vi "WPI_CameraDirect Read from Laptop.vi"(6 "Camera Settings 2":T3={"Exposure"=enum."Auto", "Exposure (%)"=50.0, "Brightness"=50, "White Balance"=enum."Auto", "Color Temp (K)"=0.0} {"Brightness" min=0 max=100}, 7 "Operation":enum16{"Read", "Reopen", "Close"}(ring), 8 "error in":errorcluster, 9 "Camera Settings":T5={"fps"=30, "compression"=30, "Image Size"=enum."320x240", "Config Shown"=FALSE}, 10 "Image":T4, 11 "address":string="10.te.am.11") -> (0 "error out":errorcluster, 2 "Image Out":T4)   [LabVIEW 2017]
doc: "This VI is intended for testing, examples, and demos. It assumes the camera is directly accssible from the computer and not the robot. It retrieves an image from either a USB or IP Axis camera.\n\nThis software is licensed. Open the labview\\readme\\WPI Robotics Library Open Source License.txt file for more information."
uses:
  <vilib>/picture/picture.llb/imagedata.ctl
  <vilib>/vision/driver/NI_Vision_Acquisition_Software.lvlib
  <vilib>/Rock Robotics/WPI/Camera/WPI_CameraDevRef.ctl
  <vilib>/Rock Robotics/WPI/Camera/WPI_CameraImageSize.ctl
  <vilib>/Rock Robotics/WPI/Camera/WPI_CameraSettings Read MJPG.ctl
  <vilib>/Rock Robotics/WPI/Camera/WPI_CameraRegistryActions.ctl
  <vilib>/Rock Robotics/WPI/Camera/WPI_CameraWhite Balance Values.ctl
  <vilib>/Rock Robotics/WPI/Camera/WPI_CameraExposure Values.ctl
  <vilib>/vision/Image Controls.llb/IMAQ Image.ctl
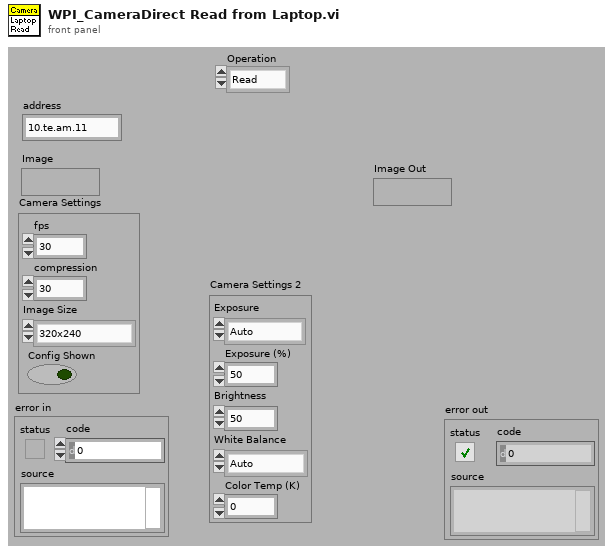
[diagram p1: front panel]
types:
  T1 = typedef "WPI_CameraExposure Values.ctl" = enum16{"Auto", "Flicker-free 50 Hz", "Flicker-free 60 Hz", "Hold current", "Custom"}
  T2 = typedef "WPI_CameraWhite Balance Values.ctl" = enum16{"Auto", "Fixed indoor", "Fixed outdoor 1", "Fixed outdoor 2", "Fixed fluorescent 1", "Fixed fluorescent 2", "Hold current", "Custom"}
  T3 = cluster{"Exposure":T1, "Exposure (%)":dbl, "Brightness":i32, "White Balance":T2, "Color Temp (K)":dbl}
  T4 = typedef "IMAQ Image.ctl" = refnum<image>
  T5 = typedef "WPI_CameraSettings Read MJPG.ctl" = cluster{"fps":i32, "compression":i32, "Image Size":T6, "Config Shown":bool}
  T6 = typedef "WPI_CameraImageSize.ctl" = enum16{"640x480", "320x240", "160x120", "Custom"}
  T7 = typedef "WPI_CameraDevRef.ctl" = cluster{"Camera Address":string, "CameraStatus":errorcluster}
  T8 = typedef "WPI_CameraRegistryActions.ctl" = enum16{"Open", "Close"}
  T9 = typedef "IMAQdx.ctl" = refnum<k21>
  T10 = cluster{"fps":bool, "compression":bool, "Image Size":bool, "Config Shown":bool}
  T11 = cluster{"Exposure":bool, "Exposure (%)":bool, "Brightness":bool, "White Balance":bool, "Color Temp (K)":bool}
  T12 = typedef "imagedata.ctl" = cluster{"image type":i32, "image depth":i32, "image":u8[], "mask":u8[], "colors":u32[], "Rectangle":cluster{"left":i16, "top":i16, "right":i16, "bottom":i16}}
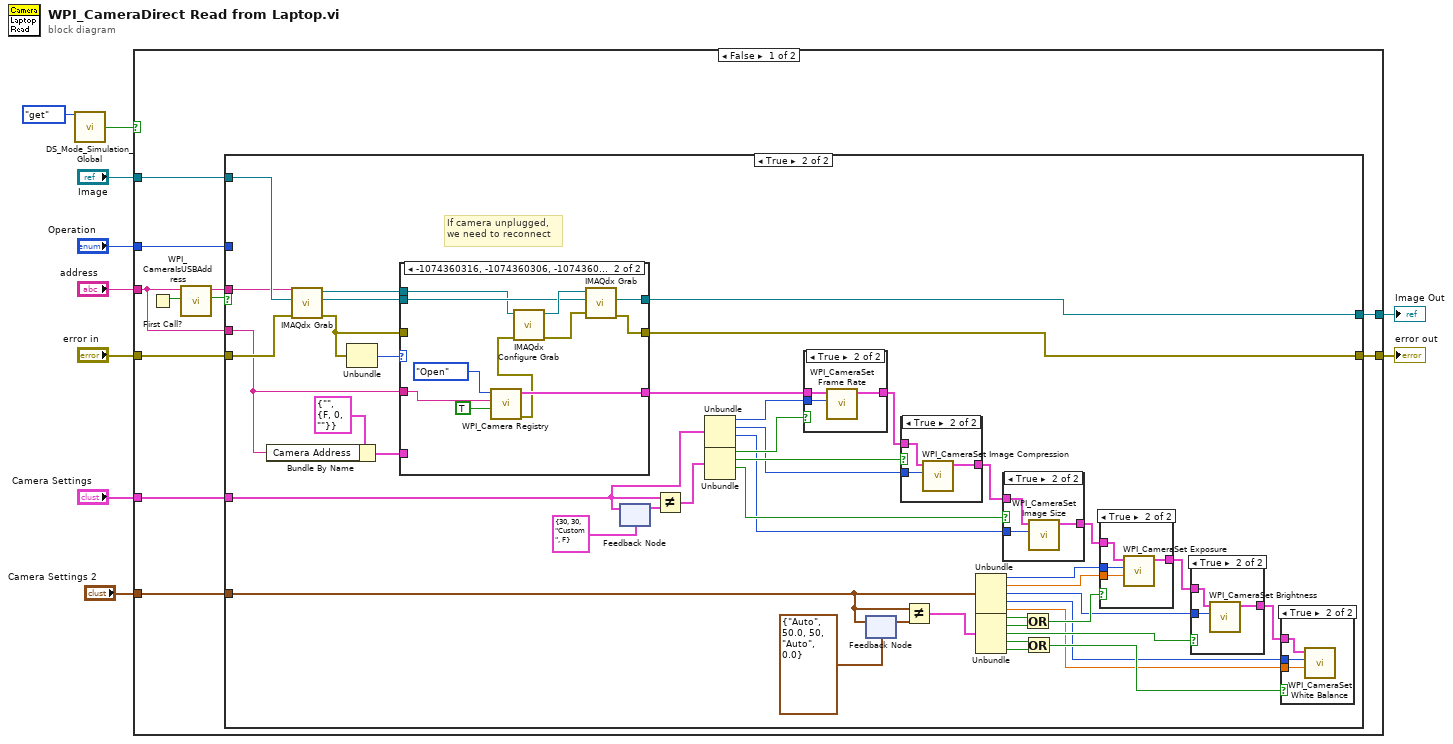
[diagram p0: block diagram]
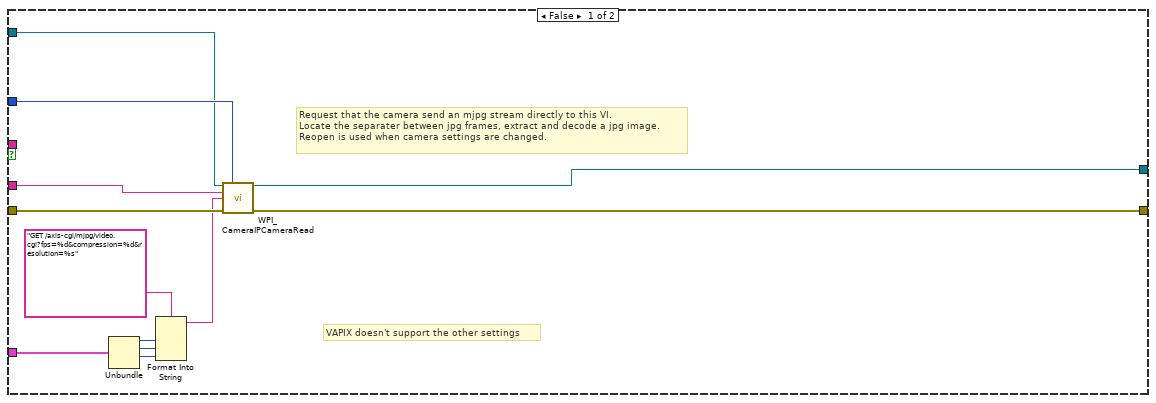
[diagram p2: hidden frame]
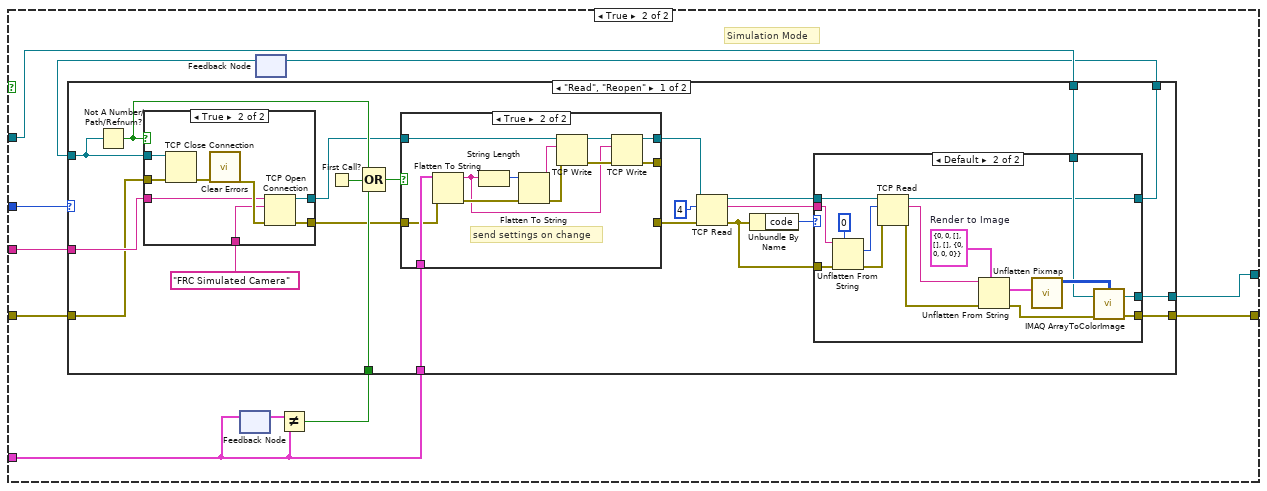
[diagram p10: hidden frame]
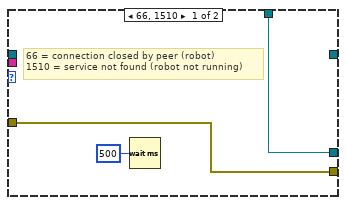
[diagram p12: hidden frame]
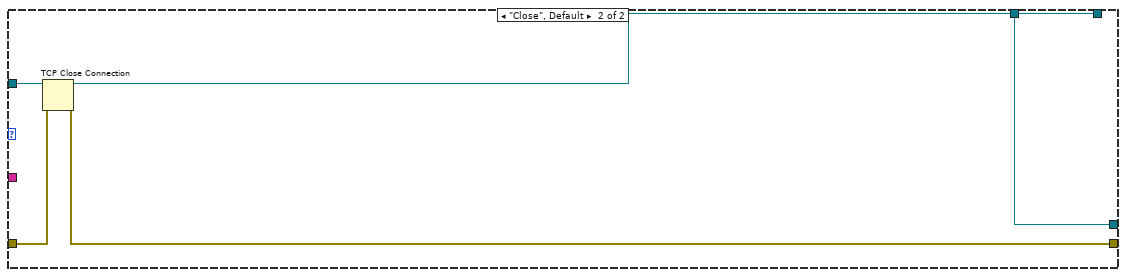
[diagram p14: hidden frame]
diagram:
  n1 = call <vilib>:"DS_Mode_Simulation_Global.vi"("menu"=enum16{"set", "get"}."get") -> ("simulated? out"=w5:bool)  [unwired: 13 in, 1 out]
  n2 = case shown="False" w5 {
    tunnel: "error in" -> [w21 w124]
    tunnel: "address" -> [w15 w125]
    tunnel: [w20 w123] -> w8
    tunnel: [w19 w122] -> w3
    tunnel: "Operation" -> [w18 w120]
    tunnel: "Image" -> [w17 w121]
    tunnel: "Camera Settings" -> [w16 w117]
    tunnel: "Camera Settings 2" -> [w11 _]
    frame False {
      n3 = First Call?() -> (First Call?: T/F=w12:bool)
      n4 = call <vilib>:"WPI_CameraIsUSBAddress.vi"("Enumerate?"=w12, "Camera Address In"=w15) -> ("USB?"=w14:bool, "Camera Address Out"=w13:string)  [unwired: 7 in, 1 out]
      n5 = case shown="True" w14 {
        tunnel: w21 -> [w31 w73]
        tunnel: w15 -> [w30 w55]
        tunnel: [w28 w70] -> w20
        tunnel: [w29 w71] -> w19
        tunnel: w18 -> [w33 _]
        tunnel: w17 -> [w32 w74]
        tunnel: w16 -> [w27 w66]
        tunnel: w13 -> [_ w58]
        tunnel: w11 -> [_ w34]
        frame False {
          # "VAPIX doesn't support the other settings"
          # "Request that the camera send an mjpg stream directly to this VI.\nLocate the separater between jpg frames, extract and decode a jpg image.\nReopen is used when camera settings are changed."
          n6 = Unbundle(w27) -> ("fps"=w24:i32, "compression"=w23:i32, "Image Size"=w22:T6)  [unwired: 1 out]
          n7 = Format Into String(format string="GET /axis-cgi/mjpg/video.cgi?fps=%d&compression=%d&resolution=%s", w24, w23, w22) -> (resulting string=w25:string)  [unwired: 2 in, 1 out]
          n8 = call <vilib>:"WPI_CameraIPCameraRead.vi"("Refnum in"=w32, "Operation"=w33, "address"=w30, "cgi string"=w25, "error in (no error)"=w31) -> ("Refnum out"=w28:T4, "error out"=w29:errorcluster)  [unwired: 6 in, 3 out]
        }
        frame True {
          # "If camera unplugged,\nwe need to reconnect"
          n9 = Bundle By Name(cluster=T7 {"Camera Address"="", "CameraStatus"={"status"=FALSE, "code"=0, "source"=""}} ("CameraDevRef"), "Camera Address"=w55) -> (w54:T7)
          n10 = call <vilib>:"IMAQdx Grab.vi"("error in"=w73, "Image In"=w74, "Session In"=w58) -> ("error out"=w72:errorcluster, "Image Out"=w75:T4, "Session Out"=w76:T9)  [unwired: 5 in, 1 out]
          n11 = Unbundle(w72) -> ("code"=w77:i32)  [unwired: 2 out]
          n12 = case shown="-1074360316, -1074360306, -1074360293" w77 {
            tunnel: [w103 w114] -> w71
            tunnel: w75 -> [w104 w111]
            tunnel: [w104 w112] -> w70
            tunnel: w76 -> [_ w106]
            tunnel: w72 -> [w103 _]
            tunnel: w55 -> [_ w108]
            tunnel: [w102 w110] -> w53
            tunnel: w54 -> [w102 _]
            frame 0, Default {
            }
            frame -1074360316, -1074360306, -1074360293 {
              n13 = call <vilib>:"WPI_Camera Registry.vi"(9:TRUE ("Disallow Simulation"), "Camera Address"=w108, "Action"=WPI_CameraRegistryActions."Open" ("Enum")) -> ("error out"=w105:errorcluster, "CameraDevRef"=w110:T7)  [unwired: 7 in]
              n14 = call <vilib>:"IMAQdx Configure Grab.vi"("error in"=w105, "Session In"=w106) -> ("error out"=w115:errorcluster, "Session Out"=w113:T9)  [unwired: 8 in]
              n15 = call <vilib>:"IMAQdx Grab.vi"("error in"=w115, "Image In"=w111, "Session In"=w113) -> ("error out"=w114:errorcluster, "Image Out"=w112:T4)  [unwired: 5 in, 2 out]
            }
          }
          n16 = feedback #1(T5 {"fps"=30, "compression"=30, "Image Size"=enum."Custom", "Config Shown"=FALSE} ("Camera Settings")) -> (w69:T5)
          n17 = feedback-in #1(w66) -> ()
          n18 = Not Equal?(x=w66, y=w69) -> (x != y?=w68:T10)
          n19 = Unbundle(w66) -> ("fps"=w61:i32, "compression"=w62:i32, "Image Size"=w63:T6)  [unwired: 1 out]
          n20 = Unbundle(w68) -> ("fps"=w67:bool, "compression"=w65:bool, "Image Size"=w64:bool)  [unwired: 1 out]
          n21 = case shown="True" w67 {
            tunnel: w61 -> [_ w101]
            tunnel: w53 -> [w98 w100]
            tunnel: [w98 w99] -> w60
            frame False {
            }
            frame True {
              n22 = call <vilib>:"WPI_CameraSet Frame Rate.vi"("Frame Rate (fps)"=w101, "CameraDevRef"=w100) -> ("CameraDevRef Out"=w99:T7)  [unwired: 8 in, 1 out]
            }
          }
          n23 = feedback #2(T3 {"Exposure"=enum."Auto", "Exposure (%)"=50.0, "Brightness"=50, "White Balance"=enum."Auto", "Color Temp (K)"=0.0} ("Camera Settings 2")) -> (w51:T3)
          n24 = feedback-in #2(w34) -> ()
          n25 = case shown="True" w65 {
            tunnel: w62 -> [_ w97]
            tunnel: w60 -> [w94 w96]
            tunnel: [w94 w95] -> w59
            frame False {
            }
            frame True {
              n26 = call <vilib>:"WPI_CameraSet Image Compression.vi"("Compression"=w97, "CameraDevRef"=w96) -> ("CameraDevRef Out"=w95:T7)  [unwired: 8 in, 1 out]
            }
          }
          n27 = Not Equal?(x=w34, y=w51) -> (x != y?=w50:T11)
          n28 = Unbundle(w34) -> ("Exposure"=w45:T1, "Exposure (%)"=w44:dbl, "Brightness"=w42:i32, "White Balance"=w36:T2, "Color Temp (K)"=w35:dbl)
          n29 = Unbundle(w50) -> ("Exposure"=w48:bool, "Exposure (%)"=w47:bool, "Brightness"=w41:bool, "White Balance"=w39:bool, "Color Temp (K)"=w38:bool)
          n30 = case shown="True" w64 {
            tunnel: w63 -> [_ w93]
            tunnel: w59 -> [w90 w92]
            tunnel: [w90 w91] -> w49
            frame False {
            }
            frame True {
              n31 = call <vilib>:"WPI_CameraSet Image Size.vi"("Image Size"=w93, "CameraDevRef"=w92) -> ("CameraDevRef Out"=w91:T7)  [unwired: 8 in, 1 out]
            }
          }
          n32 = Or(x=w48, y=w47) -> (x .or. y?=w46:bool)
          n33 = Or(x=w39, y=w38) -> (x .or. y?=w37:bool)
          n34 = case shown="True" w46 {
            tunnel: w49 -> [w85 w89]
            tunnel: [w85 w88] -> w43
            tunnel: w45 -> [_ w87]
            tunnel: w44 -> [_ w86]
            frame False {
            }
            frame True {
              n35 = call <vilib>:"WPI_CameraSet Exposure.vi"("Exposure (%)"=w86, "Exposure"=w87, "CameraDevRef"=w89) -> ("CameraDevRef Out"=w88:T7)  [unwired: 7 in, 1 out]
            }
          }
          n36 = case shown="True" w41 {
            tunnel: w43 -> [w81 w84]
            tunnel: [w81 w83] -> w40
            tunnel: w42 -> [_ w82]
            frame False {
            }
            frame True {
              n37 = call <vilib>:"WPI_CameraSet Brightness.vi"("Brightness"=w82, "CameraDevRef"=w84) -> ("CameraDevRef Out"=w83:T7)  [unwired: 8 in, 1 out]
            }
          }
          n38 = case shown="True" w37 {
            tunnel: w40 -> [_ w80]
            tunnel: w36 -> [_ w79]
            tunnel: w35 -> [_ w78]
            frame False {
            }
            frame True {
              n39 = call <vilib>:"WPI_CameraSet White Balance.vi"("Color Temp (K)"=w78, "White Balance"=w79, "CameraDevRef"=w80) -> ()  [unwired: 7 in, 2 out]
            }
          }
        }
      }
    }
    frame True {
      # "Simulation Mode"
      n40 = feedback-in #3(w117) -> ()
      n41 = feedback #3() -> (w118:T5)  [unwired: 1 in]
      n42 = feedback #4() -> (w126:refnum<k5>)  [unwired: 1 out]
      n43 = Not Equal?(x=w118, y=w117) -> (x != y?=w116:bool)
      n44 = case shown="\"Read\", \"Reopen\"" w120 {
        tunnel: w126 -> [w148 w196]
        tunnel: w125 -> [w147 _]
        tunnel: w124 -> [w146 w195]
        tunnel: [w145 w193] -> w123
        tunnel: [w138 w194] -> w122
        tunnel: w121 -> [w144 w193]
        tunnel: w117 -> [w131 _]
        tunnel: [w139 w192] -> w119
        tunnel: w116 -> [w135 _]
        frame "Read", "Reopen" {
          n45 = Not A Number/Path/Refnum?(number/path/refnum=w148) -> (NaN/Path/Refnum?=w134:bool)
          n46 = case shown="True" w134 {
            tunnel: w148 -> [w183 w191]
            tunnel: w147 -> [_ w185]
            tunnel: [w183 w188] -> w133
            tunnel: w146 -> [w182 w187]
            tunnel: [w182 w186] -> w130
            tunnel: "FRC Simulated Camera" ("service name") -> [_ w184]
            frame False {
            }
            frame True {
              n47 = TCP Close Connection(connection ID=w191, error in (no error)=w187) -> (error out=w190:errorcluster)  [unwired: 2 out]
              n48 = call <vilib>:"Clear Errors.vi"("error in (no error)"=w190) -> ("error out"=w189:errorcluster)  [unwired: 1 in, 5 out]
              n49 = TCP Open Connection(address=w185, remote port or service name=w184, error in (no error)=w189) -> (connection ID=w188:refnum<k5>, error out=w186:errorcluster)  [unwired: 2 in]
            }
          }
          n50 = First Call?() -> (First Call?: T/F=w137:bool)
          n51 = Compound Arithmetic op=OR(w134, w137, w135) -> (w136:bool)
          n52 = case shown="True" w136 {
            tunnel: w133 -> [w150 w162]
            tunnel: w131 -> [_ w160]
            tunnel: [w150 w153] -> w132
            tunnel: w130 -> [w149 w152]
            tunnel: [w149 _] -> w129
            tunnel: [_ w151] -> _
            frame False {
            }
            frame True {
              # "send settings on change"
              n53 = Flatten To String(anything=w160, error in (no error)=w152) -> (data string=w154:string, error out=w156:errorcluster)  [unwired: 2 in, 1 out]
              n54 = String Length(string=w154) -> (length=w161:i32)
              n55 = Flatten To String(anything=w161, error in (no error)=w156) -> (data string=w159:string, error out=w157:errorcluster)  [unwired: 2 in, 1 out]
              n56 = TCP Write(connection ID=w162, data in=w159, error in (no error)=w157) -> (connection ID out=w155:refnum<k5>, error out=w158:errorcluster)  [unwired: 1 in, 1 out]
              n57 = TCP Write(connection ID=w155, data in=w154, error in (no error)=w158) -> (connection ID out=w153:refnum<k5>, error out=w151:errorcluster)  [unwired: 1 in, 1 out]
            }
          }
          n58 = TCP Read(connection ID=w132, bytes to read=4, error in (no error)=w129) -> (connection ID out=w141:refnum<k5>, data out=w142:string, error out=w128:errorcluster)  [unwired: 1 in, 1 out]
          n59 = Unbundle By Name(w128) -> ("code"=w140:i32)
          n60 = case shown="Default" w140 {
            tunnel: [w165 w177] -> w145
            tunnel: [w164 w166] -> w138
            tunnel: w144 -> [w165 w176]
            tunnel: w142 -> [_ w175]
            tunnel: w141 -> [_ w174]
            tunnel: w128 -> [w164 w172]
            tunnel: [_ w167] -> w139
            frame 66, 1510 {
              # "66 = connection closed by peer (robot)\n1510 = service not found (robot not running)"
              n61 = Wait (ms)(milliseconds to wait=u32 500) -> ()  [unwired: 1 out]
            }
            frame Default {
              w179 = T12 {"image type"=0, "image depth"=0, "image"=[], "mask"=[], "colors"=[], "Rectangle"={"left"=0, "top"=0, "right"=0, "bottom"=0}}  # Render to Image
              n62 = Unflatten From String(type=0 ("bytes to read"), binary string=w175, error in (no error)=w172) -> (value=w170:i32, error out=w171:errorcluster)  [unwired: 2 in, 1 out]
              n63 = TCP Read(connection ID=w174, bytes to read=w170, error in (no error)=w171) -> (connection ID out=w167:refnum<k5>, data out=w178:string, error out=w169:errorcluster)  [unwired: 1 in, 1 out]
              n64 = Unflatten From String(type=w179, binary string=w178, error in (no error)=w169) -> (value=w180:T12, error out=w168:errorcluster)  [unwired: 2 in, 1 out]
              n65 = call <vilib>:"Unflatten Pixmap.vi"("image data"=w180) -> ("24-bit pixmap"=w181:u32[][])  [unwired: 4 in, 6 out]
              n66 = call "IMAQ ArrayToColorImage"("Image Pixels (U32)"=w181, "Image"=w176, "error in (no error)"=w168) -> ("Image Out"=w177:T4, "error out"=w166:errorcluster)  [unwired: 2 in]
            }
          }
        }
        frame "Close", Default {
          n67 = TCP Close Connection(connection ID=w196, error in (no error)=w195) -> (connection ID out=w192:refnum<k5>, error out=w194:errorcluster)  [unwired: 1 out]
        }
      }
      n68 = feedback-in #4(w119) -> ()
    }
  }
  "Image Out" <- w8
  "error out" <- w3
